vi "FPGAcode2 - NoForLoop.vi"() -> ()   [LabVIEW 2015]
uses:
  <vilib>/Platform/TimedLoop/XDataNode/wakeup.ctl
  <vilib>/Platform/TimedLoop/XDataNode/XDNodeRunTimeDep.lvlib
  <vilib>/Platform/TimedLoop/XDataNode/nitl_modes.ctl
  <vilib>/Platform/TimedLoop/XDataNode/timing_clust.ctl
  <vilib>/Platform/TimedLoop/XDataNode/XDataNode.xnode
  <vilib>/eio/EIONode/EIONode.xnode
  <vilib>/rvi/eio/common/nirviEmuTemplateMethod_errors.vi
panel:
  out "Del Armed":bool
  out "Armed":bool
  out "Delay":bool
  out "Plates":bool
  in  "Filter thresholds":i16[](array[numeric])
  out "Detector 3 Correlations":i16[](array[numeric])
  out "Detector 1 Correlations":i16[](array[numeric])
  in  "Reset One Shot":bool
  in  "One Shot":bool
  in  "High Charge Limit":i16
  in  "Low Charge Limit":i16
  in  "High Velocity Count":i32
  in  "Low Velocity Count":i32
  in  "High Mass Limit":i64
  in  "Low Mass Limit":i64
  in  "Mult1":fxp<+,16,7>
  out "IO Module\\AI 0":i16
  out "IO Module\\AI 1":i16
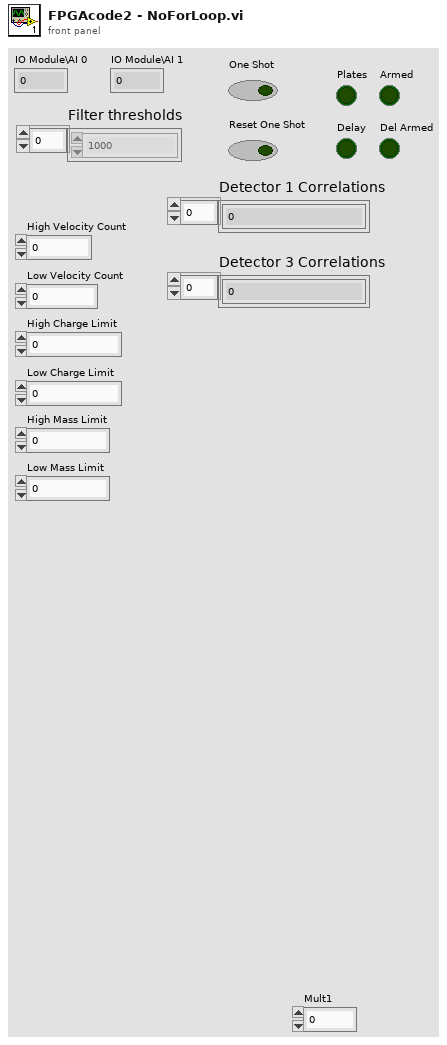
[diagram p1: front panel]
types:
  T1 = cluster{"Separation cut off 1":i32, "Filter Number":i32, "Separation cut off 2":i32}
  T2 = typedef "XDNodeRunTimeDep.lvlib/timing_clust.ctl" = cluster{"Expected End [f-1]":u64, "Actual End [f-1]":u64, "Finished Late? [f-1]":bool, "Expected End [i-1]":u64, "Actual End [i-1]":u64, "Finished Late? [i-1]":bool, "Expected Start [i]":u64, "Actual Start [i]":u64, "Expected Start [f]":u64, "Actual Start [f]":u64, "Source Name":string, "Structure Name":string, "Period":i64, "Deadline":i64, "Offset":i64, "Start":i64, "Priority":i32, "Timeout":i32, "Mode":T3, "Wakeup Reason":T4, "Error":errorcluster, "Source Type":string, "Secondary Source Type":string, "Global End Time":u64, "Global Start Time":u64, "Frame Duration":u64, "Iteration Duration":u64, "Assigned CPU":i32, "I/O Scan Engine Mode":u32}
  T3 = typedef "XDNodeRunTimeDep.lvlib/nitl_modes.ctl" = enum32{"No Change", "Process missed periods, maintain original phase", "Discard missed periods, maintain original phase", "Process missed periods, ignore original phase", "Discard missed periods, ignore original phase"}
  T4 = typedef "XDNodeRunTimeDep.lvlib/wakeup.ctl" = enum32{"Normal", "Aborted", "Asynchronous wakeup", "Timing source error", "Timed loop error", "Timeout"}
  T5 = cluster{"Old Average":i32, "New Average":i32, "Current State":u8, "Detector 1 Correlation":i32, "Detector 3 Correlation":i32, "Velocity Count":i32, "Detector Counter in":i32, "Timeout Count in":i32, "Measured Charge in":i32, "Filter Threshold":i32, "High Correlation in":i32, "Offset":i32, "Offset Average":i32, "Measured Velocity In":i32, "Mult Cluster":cluster{"Mult1":fxp<+,16,7>, "Mult1 Use?":bool}, "Final Delay Count In":u16, "Delay1 In":i32}
  T6 = cluster{"High Charge Limit":i16, "Low Charge Limit":i16, "Time Out Limit":i32, "High Velocity Count":i32, "Low Velocity Count":i32, fxp<+,30,25>, "High Mass Limit":i64, "Low Mass Limit":i64}
  T7 = cluster{"Average Out":i32, "Next State":u8, "Velocity Count out":i32, "Detector counter out":i32, "Timeout count out":u32, "Measured Charge Out":i32, "High Correlation Out":i32, "Plates":bool, "Offset Out":i32, "Measured Velocity Out":i32, "Final Delay Count Out":u16, "Out1":bool, "Delay1":i32}
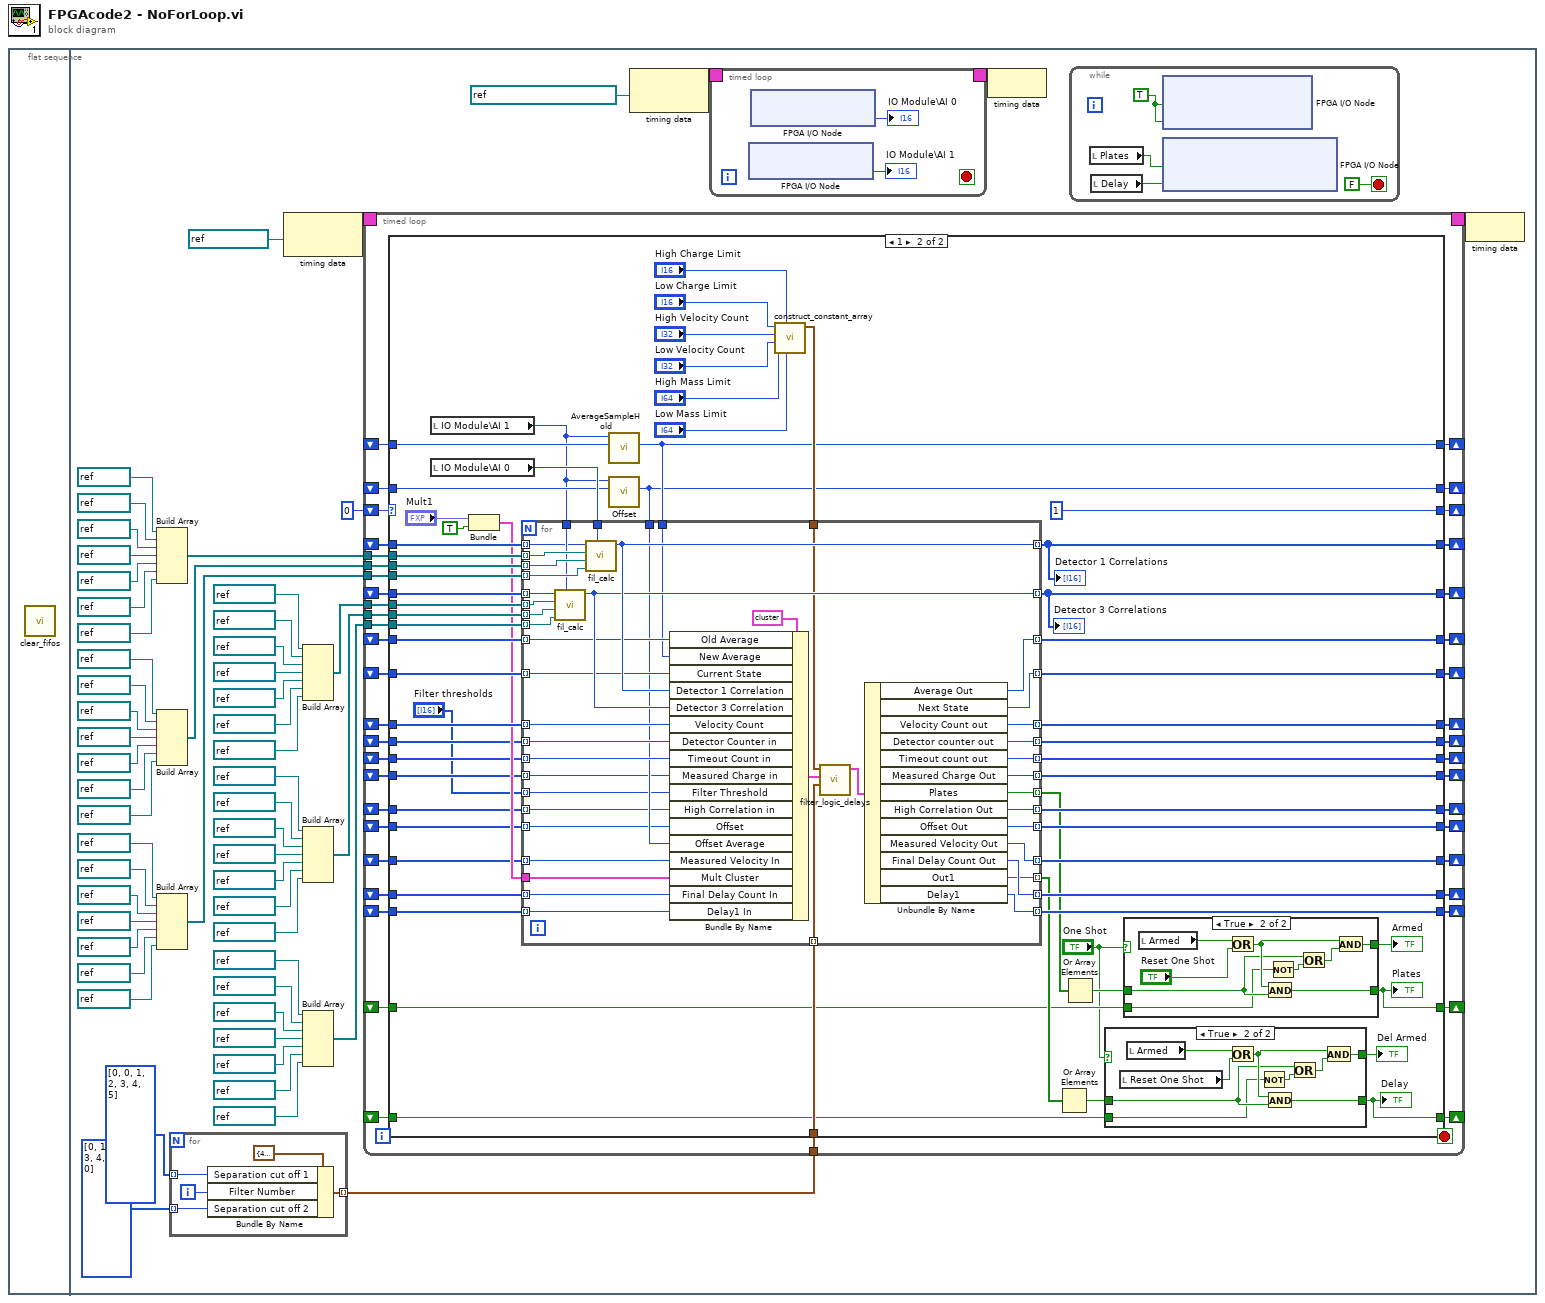
[diagram p0: block diagram]
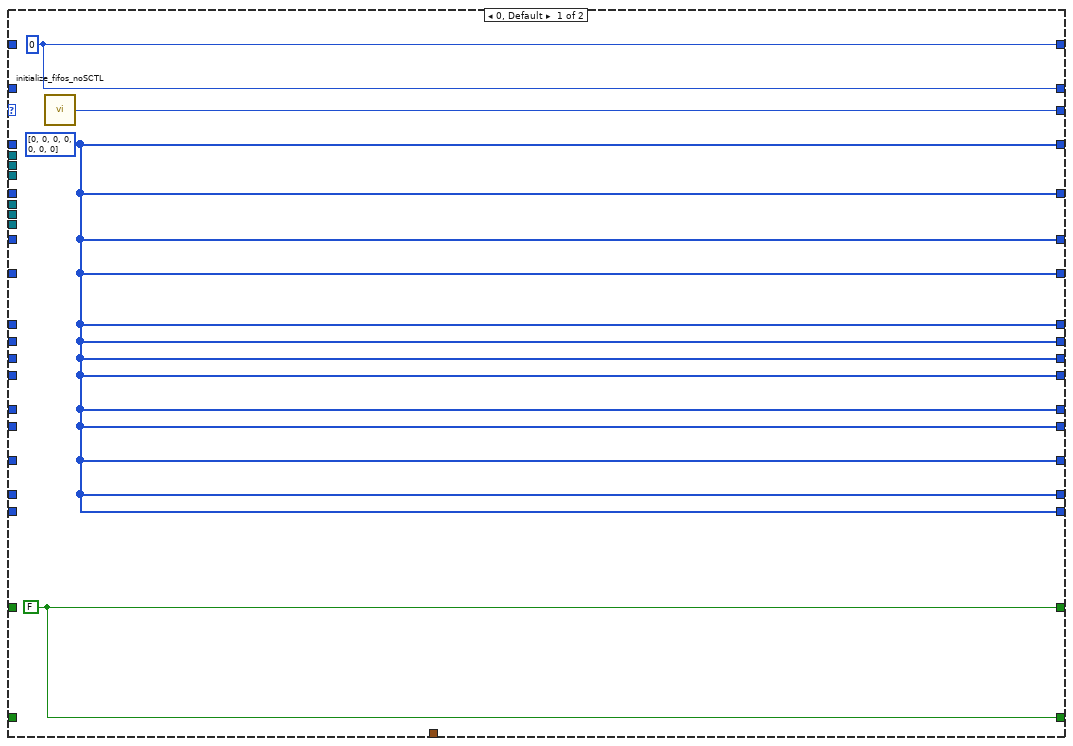
[diagram p2: hidden frame]
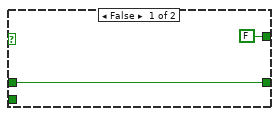
[diagram p3: hidden frame]
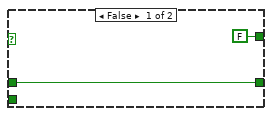
[diagram p4: hidden frame]
diagram:
  n1 = flat-sequence {
    frame #0 {
      n2 = call "clear_fifos.vi"() -> ()  [unwired: 1 in]
    }
    frame #1 {
      n3 = Build Array(refnum<k21> "fil1.1" ("FIFO 1"), refnum<k21> "fil2.1" ("FIFO 1"), refnum<k21> "fil3.1" ("FIFO 1"), refnum<k21> "fil4.1" ("FIFO 1"), refnum<k21> "fil5.1" ("FIFO 1"), refnum<k21> "fil6.1" ("FIFO 1"), refnum<k21> "fil7.1" ("FIFO 1")) -> (w51:refnum<k21>[])
      n4 = Build Array(refnum<k21> "fil1.2" ("FIFO 1"), refnum<k21> "fil2.2" ("FIFO 1"), refnum<k21> "fil3.2" ("FIFO 1"), refnum<k21> "fil4.2" ("FIFO 1"), refnum<k21> "fil5.2" ("FIFO 1"), refnum<k21> "fil6.2" ("FIFO 1"), refnum<k21> "fil7.2" ("FIFO 1")) -> (w8:refnum<k21>[])
      n5 = Build Array(refnum<k21> "fil1.3" ("FIFO 1"), refnum<k21> "fil2.3" ("FIFO 1"), refnum<k21> "fil3.3" ("FIFO 1"), refnum<k21> "fil4.3" ("FIFO 1"), refnum<k21> "fil5.3" ("FIFO 1"), refnum<k21> "fil6.3" ("FIFO 1"), refnum<k21> "fil7.3" ("FIFO 1")) -> (w7:refnum<k21>[])
      n6 = for {
        tunnel: i32[] [0, 0, 1, 2, 3, 4, 5] -> [w62] mode=indexing
        tunnel: i32[] [0, 1, 2, 3, 4, 5, 0] -> [w61] mode=indexing
        tunnel: [w59] -> w1 mode=indexing
        i -> [w60]
        n7 = Bundle By Name(cluster=T1 {"Separation cut off 1"=4, "Filter Number"=5, "Separation cut off 2"=6} ("Filter Specific Constants"), "Separation cut off 1"=w62, "Filter Number"=w60, "Separation cut off 2"=w61) -> (w59:T1)
      }
      n8 = node-c288(refnum<k21> "26.67MHz" ("Source Name")) -> (w58:T2)
      n9 = Build Array(refnum<k21> "fil1.1 2" ("FIFO 1"), refnum<k21> "fil2.1 2" ("FIFO 1"), refnum<k21> "fil3.1 2" ("FIFO 1"), refnum<k21> "fil4.1 2" ("FIFO 1"), refnum<k21> "fil5.1 2" ("FIFO 1"), refnum<k21> "fil6.1 2" ("FIFO 1"), refnum<k21> "fil7.1 2" ("FIFO 1")) -> (w6:refnum<k21>[])
      n10 = Build Array(refnum<k21> "fil1.2 2" ("FIFO 1"), refnum<k21> "fil2.2 2" ("FIFO 1"), refnum<k21> "fil3.2 2" ("FIFO 1"), refnum<k21> "fil4.2 2" ("FIFO 1"), refnum<k21> "fil5.2 2" ("FIFO 1"), refnum<k21> "fil6.2 2" ("FIFO 1"), refnum<k21> "fil7.2 2" ("FIFO 1")) -> (w5:refnum<k21>[])
      n11 = Build Array(refnum<k21> "fil1.3 2" ("FIFO 1"), refnum<k21> "fil2.3 2" ("FIFO 1"), refnum<k21> "fil3.3 2" ("FIFO 1"), refnum<k21> "fil4.3 2" ("FIFO 1"), refnum<k21> "fil5.3 2" ("FIFO 1"), refnum<k21> "fil6.3 2" ("FIFO 1"), refnum<k21> "fil7.3 2" ("FIFO 1")) -> (w4:refnum<k21>[])
      n12 = timed-loop {
        timing: w58 -> [_]
        timing-out: [_] -> w57
        shift-right: [w117] -> _
        shift-left: i16 0 ("Output State") -> [w118]
        shift-right: [w111] -> _
        shift-left: _ -> [w116]
        tunnel: w51 -> [w115]
        tunnel: w8 -> [w114]
        tunnel: w7 -> [w113]
        shift-right: [w112] -> _
        shift-left: _ -> [w110]
        tunnel: w6 -> [w109]
        tunnel: w5 -> [w108]
        tunnel: w4 -> [w107]
        tunnel: w1 -> [w106]
        shift-right: [w104] -> _
        shift-left: _ -> [w105]
        shift-right: [w102] -> _
        shift-left: _ -> [w103]
        shift-right: [w100] -> _
        shift-left: _ -> [w101]
        shift-right: [w86] -> _
        shift-left: _ -> [w99]
        shift-right: [w97] -> _
        shift-left: _ -> [w98]
        shift-right: [w95] -> _
        shift-left: _ -> [w96]
        shift-right: [w85] -> _
        shift-left: _ -> [w94]
        shift-right: [w84] -> _
        shift-left: _ -> [w93]
        shift-right: [w80] -> _
        shift-left: _ -> [w92]
        shift-right: [w90] -> _
        shift-left: _ -> [w91]
        shift-right: [w83] -> _
        shift-left: _ -> [w89]
        shift-right: [w82] -> _
        shift-left: _ -> [w88]
        shift-right: [w81] -> _
        shift-left: _ -> [w87]
        shift-right: [w79] -> _
        shift-left: _ -> [w78]
        shift-right: [w76] -> _
        shift-left: _ -> [w77]
        stop <- _ stop-if-true
        n13 = case shown="1" w118 {
          tunnel: [w122 i16 1 ("Output State")] -> w117
          tunnel: w110 -> [_ w183]
          tunnel: w116 -> [_ w182]
          tunnel: w115 -> [_ w181]
          tunnel: w114 -> [_ w180]
          tunnel: w113 -> [_ w179]
          tunnel: [w120 w174] -> w112
          tunnel: [w120 w175] -> w111
          tunnel: w109 -> [_ w178]
          tunnel: w108 -> [_ w177]
          tunnel: w107 -> [_ w176]
          tunnel: w106 -> [_ w173]
          tunnel: w105 -> [_ w172]
          tunnel: [w120 w171] -> w104
          tunnel: w103 -> [_ w170]
          tunnel: [w121 w154] -> w102
          tunnel: w101 -> [_ w167]
          tunnel: [w120 w166] -> w100
          tunnel: w99 -> [_ w165]
          tunnel: w98 -> [_ w164]
          tunnel: [w120 w163] -> w97
          tunnel: w96 -> [_ w162]
          tunnel: [w120 w161] -> w95
          tunnel: w94 -> [_ w157]
          tunnel: w93 -> [_ w156]
          tunnel: w92 -> [_ w155]
          tunnel: w91 -> [_ w153]
          tunnel: [w121 w151] -> w90
          tunnel: w89 -> [_ w150]
          tunnel: w88 -> [_ w148]
          tunnel: w87 -> [_ w147]
          tunnel: [w120 w146] -> w86
          tunnel: [w120 w145] -> w85
          tunnel: [w120 w144] -> w84
          tunnel: [w120 w143] -> w83
          tunnel: [w120 w142] -> w82
          tunnel: [w120 w141] -> w81
          tunnel: [w120 w140] -> w80
          tunnel: [w119 w134] -> w79
          tunnel: w78 -> [_ w135]
          tunnel: w77 -> [_ w131]
          tunnel: [w119 w130] -> w76
          frame 0, Default {
            w119 = FALSE
            w120 = i16[] [0, 0, 0, 0, 0, 0, 0]
            w121 = i16 0 ("Output New Average")
            n14 = call "initialize_fifos_noSCTL.vi"() -> ("Output State"=w122:i16)
          }
          frame 1 {
            n15 = local read "IO Module\\AI 1"() -> (w152:i16)
            n16 = local read "IO Module\\AI 0"() -> (w169:i16)
            n17 = Bundle("Mult1"="Mult1", TRUE) -> (w158:cluster{"Mult1":fxp<+,16,7>, bool})  [unwired: 1 in]
            n18 = call "AverageSampleHold.vi"("Previous Average"=w170, "Input Value"=w152) -> ("Output New Average"=w154:i16)  [unwired: 9 in]
            n19 = call "Offset.vi"("Previous Average"=w153, "Input Value"=w152) -> ("Output New Average"=w151:i16)  [unwired: 9 in]
            n20 = call "construct_constant_array.vi"("Low Mass Limit"="Low Mass Limit", "High Charge Limit"="High Charge Limit", "High Mass Limit"="High Mass Limit", "Low Velocity Count"="Low Velocity Count", "High Velocity Count"="High Velocity Count", "Low Charge Limit"="Low Charge Limit") -> ("constants cluster"=w168:T6)  [unwired: 5 in]
            n21 = for {
              tunnel: [w244] -> w174 mode=indexing
              tunnel: w183 -> [w235] mode=indexing
              tunnel: w182 -> [w236] mode=indexing
              tunnel: [w243] -> w175 mode=indexing
              tunnel: w181 -> [w250] mode=indexing
              tunnel: w180 -> [w251] mode=indexing
              tunnel: w179 -> [w249] mode=indexing
              tunnel: w178 -> [w248] mode=indexing
              tunnel: w177 -> [w247] mode=indexing
              tunnel: w176 -> [w246] mode=indexing
              tunnel: w173 -> [w241] mode=indexing
              tunnel: w172 -> [w238] mode=indexing
              tunnel: [w239] -> w171 mode=indexing
              tunnel: w152 -> [w237]
              tunnel: w169 -> [w234]
              tunnel: w168 -> [w233]
              tunnel: w167 -> [w232] mode=indexing
              tunnel: [w231] -> w166 mode=indexing
              tunnel: w165 -> [w230] mode=indexing
              tunnel: w164 -> [w229] mode=indexing
              tunnel: [w228] -> w163 mode=indexing
              tunnel: w162 -> [w227] mode=indexing
              tunnel: [w226] -> w161 mode=indexing
              tunnel: w158 -> [w225]
              tunnel: w157 -> [w224] mode=indexing
              tunnel: w156 -> [w223] mode=indexing
              tunnel: w155 -> [w222] mode=indexing
              tunnel: w151 -> [w221]
              tunnel: w154 -> [w220]
              tunnel: w150 -> [w219] mode=indexing
              tunnel: "Filter thresholds" -> [w218] mode=indexing
              tunnel: w148 -> [w217] mode=indexing
              tunnel: w147 -> [w216] mode=indexing
              tunnel: [w215] -> w146 mode=indexing
              tunnel: [w214] -> w145 mode=indexing
              tunnel: [w213] -> w144 mode=indexing
              tunnel: [w212] -> w143 mode=indexing
              tunnel: [w209] -> w142 mode=indexing
              tunnel: [w211] -> w141 mode=indexing
              tunnel: [w210] -> w140 mode=indexing
              tunnel: [w208] -> w139 mode=indexing
              tunnel: [w207] -> w138 mode=indexing
              n22 = call "fil_calc.vi"("AI (Current Detector Output)"=w237, "FIFO 3"=w246, "FIFO 2"=w247, "FIFO 1"=w248, "Previous Detector Correlation"=w236) -> ("Detector Correlation Out"=w243:i16)  [unwired: 5 in]
              n23 = call "fil_calc.vi"("AI (Current Detector Output)"=w234, "FIFO 3"=w249, "FIFO 2"=w251, "FIFO 1"=w250, "Previous Detector Correlation"=w235) -> ("Detector Correlation Out"=w244:i16)  [unwired: 5 in]
              n24 = Bundle By Name(cluster=T5 {"Old Average"=0, "New Average"=0, "Current State"=0, "Detector 1 Correlation"=0, "Detector 3 Correlation"=0, "Velocity Count"=0, "Detector Counter in"=0, "Timeout Count in"=0, "Measured Charge in"=0, "Filter Threshold"=0, "High Correlation in"=0, "Offset"=0, "Offset Average"=0, "Measured Velocity In"=0, "Mult Cluster"={"Mult1"=0.0, "Mult1 Use?"=FALSE}, "Final Delay Count In"=0, "Delay1 In"=0} ("Variables Cluster"), "Old Average"=w238, "New Average"=w220, "Current State"=w232, "Detector 1 Correlation"=w244, "Detector 3 Correlation"=w243, "Velocity Count"=w230, "Detector Counter in"=w224, "Timeout Count in"=w223, "Measured Charge in"=w219, "Filter Threshold"=w218, "High Correlation in"=w217, "Offset"=w216, "Offset Average"=w221, "Measured Velocity In"=w222, "Mult Cluster"=w225, "Final Delay Count In"=w227, "Delay1 In"=w229) -> (w242:T5)
              n25 = call "filter_logic_delays.vi"("Filter Specific Constants"=w241, "Variables Cluster"=w242, "controls cluster"=w233) -> ("Output Cluster"=w240:T7)  [unwired: 8 in]
              n26 = Unbundle By Name(w240) -> ("Average Out"=w239:i32, "Next State"=w231:u8, "Velocity Count out"=w215:i32, "Detector counter out"=w214:i32, "Timeout count out"=w213:u32, "Measured Charge Out"=w212:i32, "Plates"=w208:bool, "High Correlation Out"=w209:i32, "Offset Out"=w211:i32, "Measured Velocity Out"=w210:i32, "Final Delay Count Out"=w226:u16, "Out1"=w207:bool, "Delay1"=w228:i32)
            }
            "Detector 1 Correlations" <- w174
            "Detector 3 Correlations" <- w175
            n27 = Or Array Elements(Boolean array=w138) -> (logical OR=w133:bool)
            n28 = Or Array Elements(Boolean array=w139) -> (logical OR=w137:bool)
            n29 = case shown="True" "One Shot" {
              tunnel: [w186 w192] -> w130
              tunnel: w133 -> [w186 w189]
              tunnel: [FALSE w194] -> w129
              tunnel: w131 -> [_ w188]
              frame False {
              }
              frame True {
                n30 = local read "Reset One Shot"() -> (w187:bool)
                n31 = local read "Armed"() -> (w195:bool)
                n32 = Or(x=w195, y=w187) -> (x .or. y?=w193:bool)
                n33 = Not(x=w188) -> (.not. x?=w190:bool)
                n34 = And(x=w193, y=w189) -> (x .and. y?=w192:bool)
                n35 = Or(x=w189, y=w190) -> (x .or. y?=w191:bool)
                n36 = And(x=w193, y=w191) -> (x .and. y?=w194:bool)
              }
            }
            "Delay" <- w130
            "Del Armed" <- w129
            n37 = case shown="True" "One Shot" {
              tunnel: [w197 w202] -> w134
              tunnel: w137 -> [w197 w199]
              tunnel: [FALSE w204] -> w136
              tunnel: w135 -> [_ w198]
              frame False {
              }
              frame True {
                n38 = local read "Armed"() -> (w206:bool)
                n39 = Or(x=w206, y="Reset One Shot") -> (x .or. y?=w203:bool)
                n40 = And(x=w203, y=w199) -> (x .and. y?=w202:bool)
                n41 = Not(x=w198) -> (.not. x?=w200:bool)
                n42 = Or(x=w199, y=w200) -> (x .or. y?=w201:bool)
                n43 = And(x=w203, y=w201) -> (x .and. y?=w204:bool)
              }
            }
            "Plates" <- w134
            "Armed" <- w136
          }
        }
      }
      n44 = node-c288(refnum<k21> "IO Module\\Data Clock" ("Source Name")) -> (w55:T2)
      n45 = timed-loop {
        timing: w55 -> [_]
        timing-out: [_] -> w54
        stop <- _ stop-if-true
        n46 = xnode "FPGA I/O Node"() -> ("IO Module\\AI 1"=→"IO Module\\AI 1":i16)  [unwired: 1 in, 1 out]
        n47 = xnode "FPGA I/O Node"() -> ("IO Module\\AI 0"=→"IO Module\\AI 0":i16)  [unwired: 1 in, 1 out]
      }
      n48 = node-c288(w54) -> ()
      n49 = while {
        stop <- FALSE stop-if-true
        w75 = TRUE ("IO Module\\PFI Enable")
        n50 = local read "Plates"() -> (w73:bool)
        n51 = local read "Delay"() -> (w72:bool)
        n52 = xnode "FPGA I/O Node"("IO Module\\PFI 0 WE"=w75, "IO Module\\PFI 1 WE"=w75) -> ()  [unwired: 2 in, 2 out]
        n53 = xnode "FPGA I/O Node"("IO Module\\PFI 0 Wr Data"=w73, "IO Module\\PFI 1 Wr Data"=w72) -> ()  [unwired: 2 in, 2 out]
      }
      n54 = node-c288(w57) -> ()
    }
  }
